vi "lv deref string.vi"(7 "do not free":bool, 8 "error in":errorcluster, 11 "string handle":i32) -> (0 "error out":errorcluster, 2 "outbuffer":string)   [LabVIEW 2026]
uses:
  bin/nominalClient_64.dll
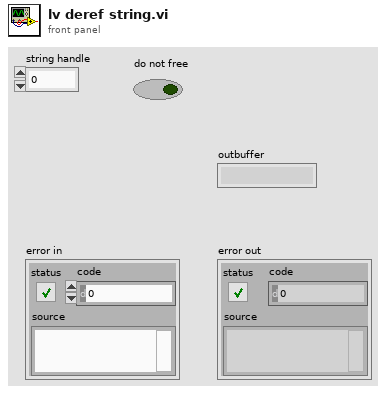
[diagram p1: front panel]
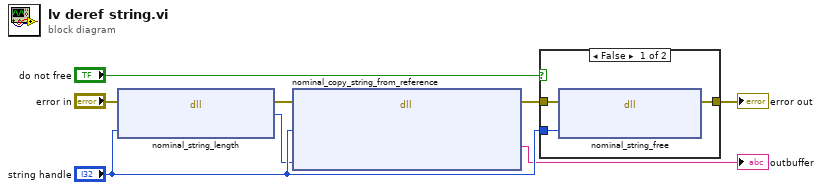
[diagram p0: block diagram]
diagram:
  n1 = dll-call lib="C:/sw/nominal-c/bin/nominalClient_64.dll" fn="nominal_string_length"(error in="error in", "string handle"="string handle") -> (error out=w2:errorcluster, "return type"=w5:u32)  [unwired: 3 in, 1 out]
  n2 = dll-call lib="C:/sw/nominal-c/bin/nominalClient_64.dll" fn="nominal_copy_string_from_reference"(error in=w2, "string handle"="string handle", "buffersize"=w5) -> (error out=w3:errorcluster, "outbuffer"=→"outbuffer":string)  [unwired: 6 in, 1 out]
  n3 = case shown="False" "do not free" {
    tunnel: "string handle" -> [w11 _]
    tunnel: [w10 w12] -> w4
    tunnel: w3 -> [w9 w12]
    frame False {
      n4 = dll-call lib="C:/sw/nominal-c/bin/nominalClient_64.dll" fn="nominal_string_free"(error in=w9, "string handle"=w11) -> (error out=w10:errorcluster)  [unwired: 4 in, 1 out]
    }
    frame True {
    }
  }
  "error out" <- w4
